vi "延时.vi"(8 "error in (no error)":errorcluster caption="错误输入（无错误）", 11 "延时（百毫秒）":i32) -> (0 "error out":errorcluster caption="错误输出")   [LabVIEW 2018]
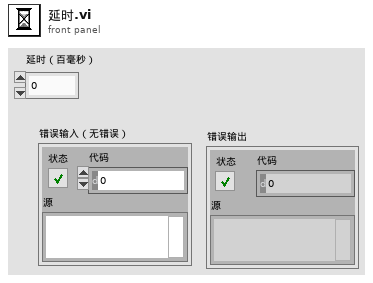
[diagram p1: front panel]
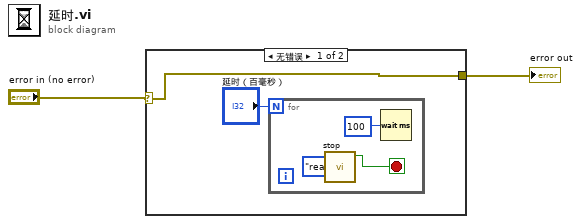
[diagram p0: block diagram]
diagram:
  n1 = case shown="无错误" "error in (no error)" {
    selector: "error in (no error)" -> [w4 w8]
    tunnel: [w4 w8] -> w1
    frame No Error {
      n2 = for {
        N: "延时（百毫秒）" -> [_]
        stop <- w5 stop-if-true
        n3 = call "stop.vi"("枚举"=enum16{"write", "read"}."read") -> ("停止"=w5:bool)  [unwired: 10 in]
        n4 = Wait (ms)(milliseconds to wait=u32 100 ("y")) -> ()  [unwired: 1 out]
      }
    }
    frame Error {
    }
  }
  "error out" <- w1
